vi "Return Plugin Interface.vi"(8 "error in (no error)":errorcluster, 9 "timeout in ms (0)":i32 format="%d ms", 10 "Plugin Interface":refnum<class "Plugin Interface.lvclass">, 11 "Plugin Interface Pool in":refnum<class "Plugin Interface Pool.lvclass">) -> (0 "error out":errorcluster, 1 "timed out?":bool, 3 "Plugin Interface Pool out":refnum<class "Plugin Interface Pool.lvclass">)   [LabVIEW 2017, in "DSF Core.lvlib" / "Plugin Interface Pool.lvclass"]
uses:
  Plugin Interface Pool.lvclass
  C:/Git/DSF/Data Sharing Framework/Source/Core/Engine/Classes/Thread Pool/Pool.lvclass
  Interfaces/Plugin/Plugin Interface.lvclass
  C:/Git/DSF/Data Sharing Framework/Source/Core/Engine/Classes/Interfaces/Interface/Interface.lvclass
  Interfaces/Interface/Interface.lvclass/Interface.ctl
  Pool.lvclass/Pool.ctl
  Pool.lvclass
  Interfaces/Interface/Interface.lvclass
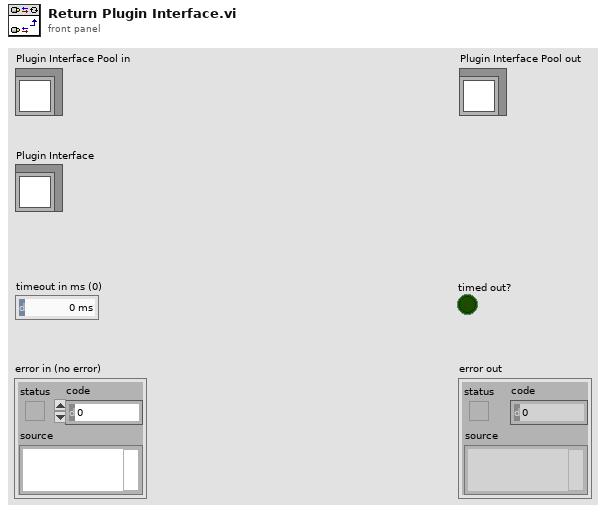
[diagram p1: front panel]
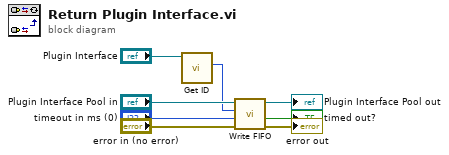
[diagram p0: block diagram]
diagram:
  n1 = call "Get ID.vi"("Interface in"="Plugin Interface") -> ("ID"=w1:i32)  [unwired: 9 in, 1 out]
  n2 = call "Write FIFO.vi"("error in (no error)"="error in (no error)", "timeout in ms (0)"="timeout in ms (0)", "element"=w1, "Pool in"="Plugin Interface Pool in") -> ("error out"=→"error out":errorcluster, "timed out?"=→"timed out?":bool, "Pool out"=→"Plugin Interface Pool out":refnum<class "Plugin Interface Pool.lvclass">)  [unwired: 5 in]
